vi "SetMonitor.vi"(6 "Inherit Monitor from Main VI? (T)":bool=TRUE, 8 "error in (no error)":errorcluster, 9 "Monitor Selection":i16) -> (0 "error out":errorcluster, 2 "Monitor":i16)   [LabVIEW 2010]
doc: "This VI is used to define the caller VI's monitor selection.\nThe default is to inherit the monitor from the main VI but if \"Inherit Monitor from Main VI\" is False then you can specify the monitor by chaning the monitor selection control"
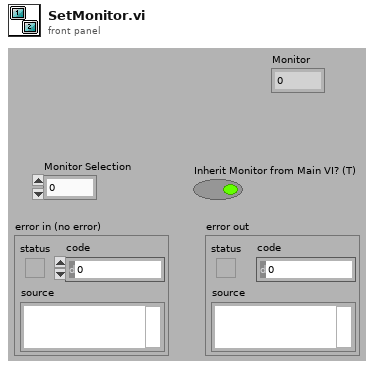
[diagram p1: front panel]
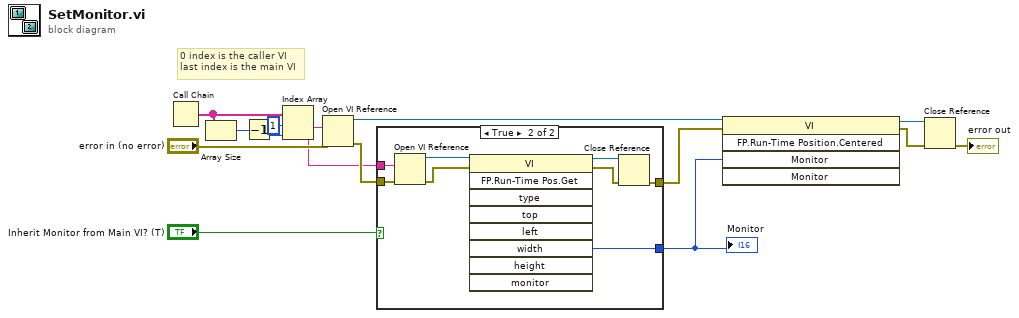
[diagram p0: block diagram]
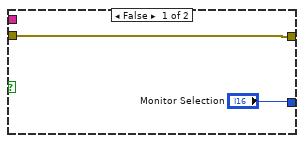
[diagram p2: hidden frame]
diagram:
  # "0 index is the caller VI\nlast index is the main VI"
  n1 = Call Chain() -> (call chain=w6:string[])
  n2 = Array Size(array=w6) -> (size(s)=w5:i32)
  n3 = Decrement(x=w5) -> (x-1=w2:i32)
  n4 = Index Array(array=w6, index #1=1 ("index"), index #2=w2) -> (element #1=w4:string, element #2=w3:string)
  n5 = Open VI Reference(vi path=w4, error in (no error)="error in (no error)") -> (vi reference=w14:refnum<vi>, error out=w8:errorcluster)  [unwired: 4 in]
  n6 = case shown="True" "Inherit Monitor from Main VI? (T)" {
    tunnel: [w16 w22] -> w15
    tunnel: ["Monitor Selection" w21] -> w13
    tunnel: w8 -> [w16 w20]
    tunnel: w3 -> [_ w18]
    frame False {
    }
    frame True {
      n7 = Open VI Reference(vi path=w18, error in (no error)=w20) -> (vi reference=w25:refnum<vi>, error out=w19:errorcluster)  [unwired: 4 in]
      n8 = invoke class="VI" method="FP.Run-Time Pos.Get"(reference=w25, error in=w19) -> (reference out=w24:refnum<vi>, error out=w23:errorcluster, "width"=w21:i16)  [unwired: 7 in, 6 out]
      n9 = Close Reference(reference=w24, error in (no error)=w23) -> (error out=w22:errorcluster)
    }
  }
  "Monitor" <- w13
  n10 = invoke class="VI" method="FP.Run-Time Position.Centered"(reference=w14, error in=w15, "Monitor"=w13) -> (reference out=w11:refnum<vi>, error out=w12:errorcluster)  [unwired: 2 in, 3 out]
  n11 = Close Reference(reference=w11, error in (no error)=w12) -> (error out=→"error out":errorcluster)
